vi "19.1.2-LCD Reader.vi"() -> ()   [LabVIEW 2017]
doc: "This example shows how to compute the histogram of an image or a region in the image. This example also shows how to set up and use the display tools to select and work on different regions in the image interactively."
uses:
  <vilib>/vision/NI_Vision_Development_Module.lvlib
panel:
  out "Output value":dbl format="%.2f"
  out "UUT":T1(plugin-control)
  out "Segments status":T2(array[cluster])
  out "Output string":string
  out "Template":T1(plugin-control)
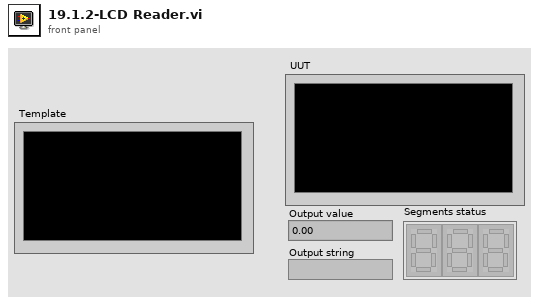
[diagram p1: front panel]
types:
  T1 = typedef "IMAQ Image.ctl" = refnum<image>
  T2 = cluster{bool, bool, bool, bool, bool, bool, bool}[]
  T3 = typedef "Image Type" = u32
  T4 = typedef "IMAQ Rectangle" = cluster{"Left":i32, "Top":i32, "Right":i32, "Bottom":i32, "Rotation":dbl}
  T5 = typedef "ROI Descriptor" = cluster{"Global Rectangle":i32[], "Contours":cluster{"ID":enum32{"External", "Internal"}, "Type":u32, "Coordinates":i32[]}[]}
  T6 = cluster{"Global Rectangle":i32[], "Contours":cluster{"ID":enum32{"External", "Internal"}, "Type":u32, "Coordinates":i32[]}[]}
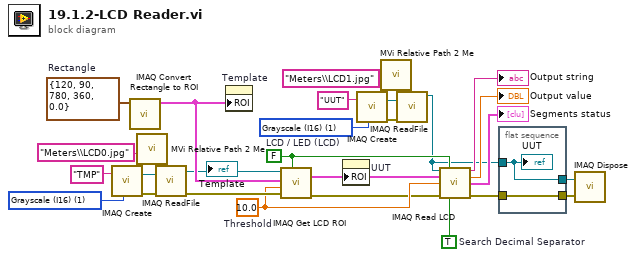
[diagram p0: block diagram]
diagram:
  w4 = T3 1 items=["Grayscale (U8)", "Grayscale (I16)", "Grayscale (SGL)", "Complex (CSG)", "RGB (U32)", "HSL (U32)", "RGB (U64)", "Grayscale (U16)"] ("Image Type")
  w12 = 10.0  # Threshold
  w11 = FALSE  # LCD / LED (LCD)
  w20 = TRUE  # Search Decimal Separator
  w21 = T4 {"Left"=120, "Top"=90, "Right"=780, "Bottom"=360, "Rotation"=0.0}  # Rectangle
  w23 = T3 1 items=["Grayscale (U8)", "Grayscale (I16)", "Grayscale (SGL)", "Complex (CSG)", "RGB (U32)", "HSL (U32)", "RGB (U64)", "Grayscale (U16)"] ("Image Type")
  n1 = call "IMAQ Create"("Image Name"="TMP", "Image Type"=w23) -> ("New Image"=w28:T1, "error out"=w27:errorcluster)  [unwired: 3 in]
  n2 = call "IMAQ Convert Rectangle to ROI"("Rectangle"=w21) -> ("ROI Descriptor"=w13:T5)  [unwired: 8 in, 1 out]
  n3 = call "MVi Relative Path 2 Me.vi"("Relative Path"="Meters\\LCD0.jpg") -> ("Appended Dir"=w25:path)  [unwired: 5 in, 1 out]
  n4 = call "IMAQ ReadFile"("File Path"=w25, "error in (no error)"=w27, "Image"=w28) -> ("error out"=w14:errorcluster, "Image Out"=w2:T1)  [unwired: 4 in, 3 out]
  "Template" <- w2
  n5 = property on="Template" class="ImageControl"("ROI"=w13) -> ()  [unwired: 2 in, 2 out]
  n6 = call "IMAQ Get LCD ROI"("LCD / LED (LCD)"=w11, "error in (no error)"=w14, "Threshold"=w12, "ROI Descriptor"=w13, "Image"=w2) -> ("error out"=w10:errorcluster, "ROI Descriptor out"=w3:T6)  [unwired: 5 in]
  n7 = property on="UUT" class="ImageControl"("ROI"=w3) -> ()  [unwired: 2 in, 2 out]
  n8 = call "IMAQ Create"("Image Name"="UUT", "Image Type"=w4) -> ("New Image"=w5:T1, "error out"=w6:errorcluster)  [unwired: 3 in]
  n9 = call "MVi Relative Path 2 Me.vi"("Relative Path"="Meters\\LCD1.jpg") -> ("Appended Dir"=w8:path)  [unwired: 5 in, 1 out]
  n10 = call "IMAQ ReadFile"("File Path"=w8, "error in (no error)"=w6, "Image"=w5) -> ("Image Out"=w1:T1)  [unwired: 4 in, 4 out]
  n11 = call "IMAQ Read LCD"("Image"=w1, "LCD/LED (LCD)"=w11, "ROI Descriptor"=w3, "Threshold"=w12, "error in (no error)"=w10, "Search Decimal Separator"=w20) -> ("Output string"=→"Output string":string, "Output value"=→"Output value":dbl, "Segments status"=→"Segments status":T2, "error out"=w16:errorcluster)  [unwired: 6 in]
  n12 = flat-sequence {
    tunnel: w1 -> [w29]
    tunnel: [w29] -> w17
    tunnel: w16 -> [w30]
    tunnel: [w30] -> w15
    frame #0 {
      "UUT" <- w29
    }
  }
  n13 = call "IMAQ Dispose"("Image"=w17, "error in (no error)"=w15) -> ()  [unwired: 4 in, 1 out]
